vi "3_loop.vi"(11 "文字列入力":string) -> (3 "文字列出力":string)   [LabVIEW 2019]
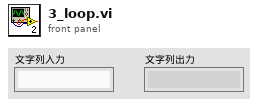
[diagram p1: front panel]
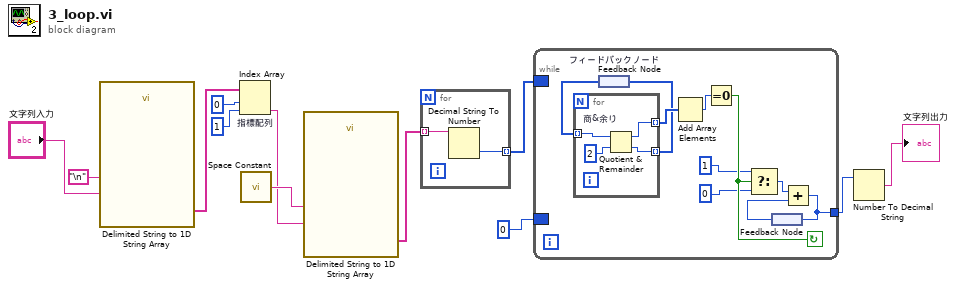
[diagram p0: block diagram]
diagram:
  n1 = call <vilib>:"Delimited String to 1D String Array.vi"("delimiter"="\n", "delimited string"="文字列入力") -> ("string array"=w7:string[])  [unwired: 9 in]
  n2 = Index Array "指標配列"(array=w7, index #1=0, index #2=1) -> (element #2=w8:string)  [unwired: 1 out]
  n3 = call <vilib>:"Space Constant.vi"() -> ("String"=w9:string)
  n4 = call <vilib>:"Delimited String to 1D String Array.vi"("delimiter"=w9, "delimited string"=w8) -> ("string array"=w10:string[])  [unwired: 9 in]
  n5 = for {
    tunnel: w10 -> [w14] mode=indexing
    tunnel: [w13] -> w2 mode=indexing
    n6 = Decimal String To Number(string=w14) -> (number=w13:i32)  [unwired: 2 in, 1 out]
  }
  n7 = while {
    tunnel: [w16] -> w11
    border: w2 -> [_]
    border: 0 -> [_]
    stop <- w22 continue-if-true
    n8 = feedback #1 "フィードバックノード"() -> (w17:i32[])
    n9 = for {
      tunnel: w17 -> [w28] mode=indexing
      tunnel: [w26] -> w18 mode=indexing
      tunnel: [w25] -> w24 mode=indexing
      n10 = Quotient & Remainder "商&余り"(x=w28, y=2) -> (x-y*floor(x/y)=w25:i32, floor(x/y)=w26:i32)
    }
    n11 = feedback-in #1(w18) -> ()
    n12 = Add Array Elements(numeric array=w24) -> (sum=w23:i32)
    n13 = Equal To 0?(x=w23) -> (x = 0?=w22:bool)
    n14 = Select(t=1, s=w22, f=0) -> (s? t:f=w19:i32)
    n15 = feedback #2 ("フィードバックノード")() -> (w15:i32)
    n16 = Add(x=w19, y=w15) -> (x+y=w16:i32)
    n17 = feedback-in #2(w16) -> ()
  }
  n18 = Number To Decimal String(number=w11) -> (decimal integer string=→"文字列出力":string)  [unwired: 1 in]
